vi "GetDevices.vi"(8 "error in (no error)":errorcluster, 11 "service":refnum<class "IcmMessageService.lvclass">) -> (0 "error out":errorcluster, 3 "Body":T1)   [LabVIEW 2016]
doc: "Queries for all equipment asset nodes, which means they have operating states."
uses:
  <vilib>/addons/InsightCM/MessageBus/MessageService/IcmMessageService.lvclass
  <vilib>/addons/InsightCM/MessageBus/Base/controls/KeyValuePair.ctl
  <vilib>/addons/InsightCM/MessageBus/Base/controls/DataGroup.ctl
  <vilib>/addons/InsightCM/MessageBus/Base/controls/DeviceState.ctl
  <vilib>/addons/InsightCM/MessageBus/Base/controls/Condition.ctl
  <vilib>/addons/InsightCM/MessageBus/Base/controls/Trigger.ctl
  <vilib>/addons/InsightCM/MessageBus/Base/controls/BurstModeTrigger.ctl
  <vilib>/addons/InsightCM/MessageBus/Base/controls/Device.ctl
  <vilib>/addons/InsightCM/MessageBus/MessageLibrary/AssetManager/controls/AssetMgrGetDeviceListResponseBody.ctl
panel:
  out "string":string
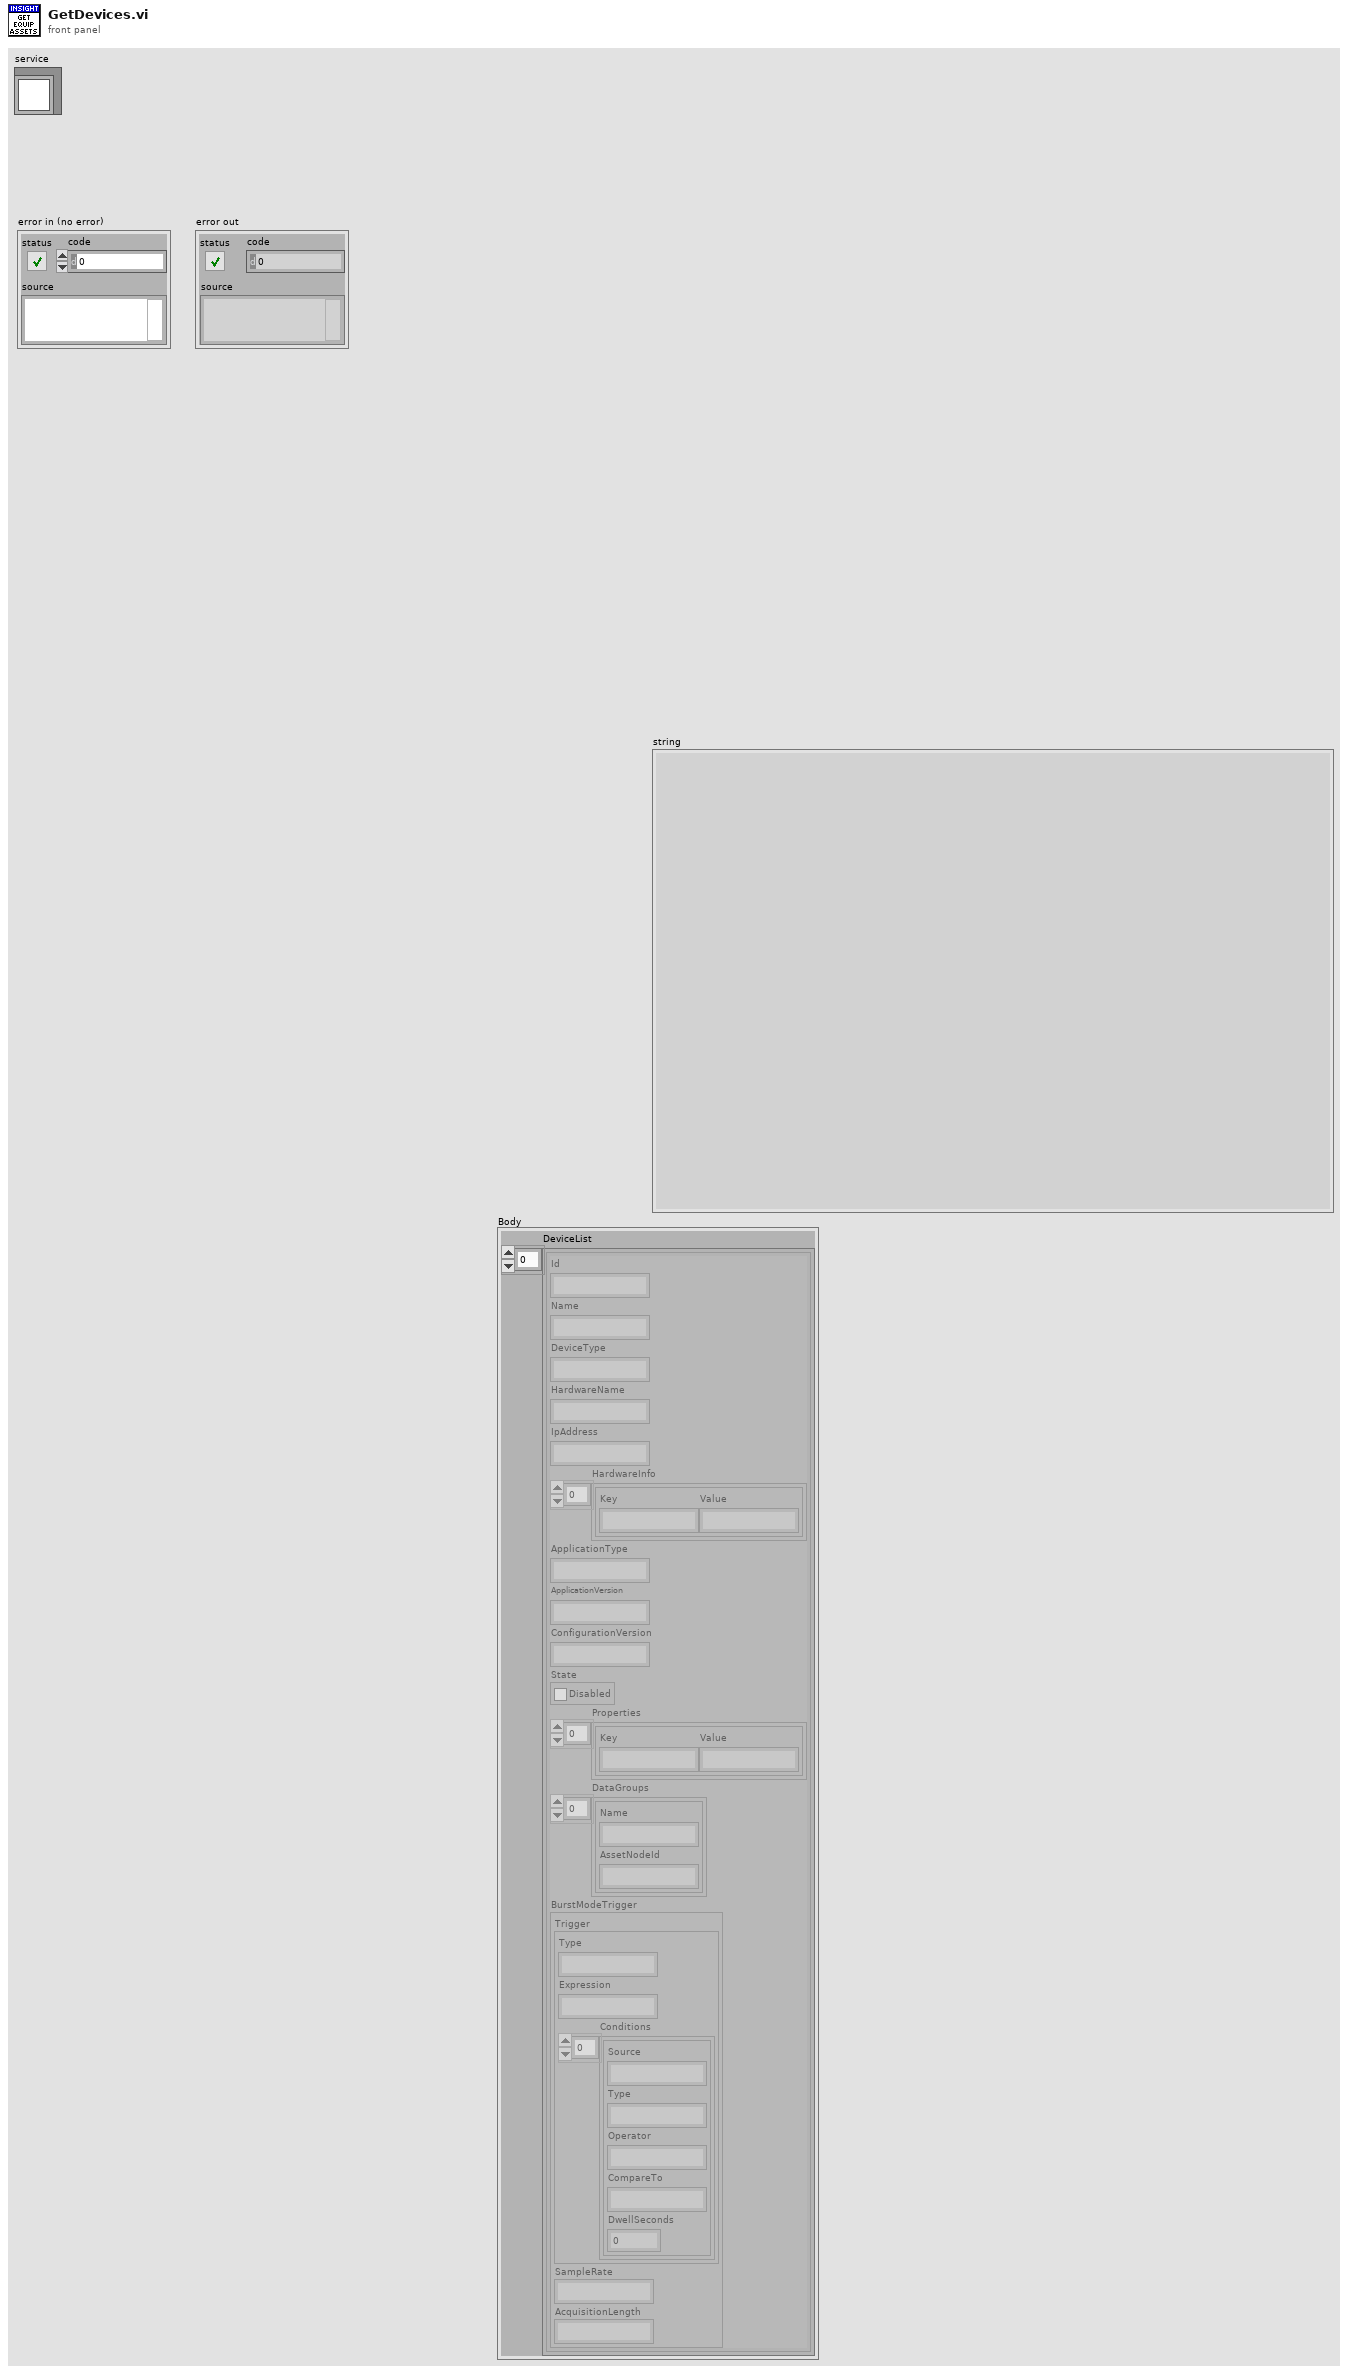
[diagram p1: front panel]
types:
  T1 = typedef "AssetMgrGetDeviceListResponseBody.ctl" = cluster{"DeviceList":T2[]}
  T2 = typedef "Device.ctl" = cluster{"Id":string, "Name":string, "DeviceType":string, "HardwareName":string, "IpAddress":string, "HardwareInfo":T3[], "ApplicationType":string, "ApplicationVersion":string, "ConfigurationVersion":string, "State":T4, "Properties":T3[], "DataGroups":T5[], "BurstModeTrigger":T6}
  T3 = typedef "KeyValuePair.ctl" = cluster{"Key":string, "Value":string}
  T4 = typedef "DeviceState.ctl" = cluster{"Disabled":bool}
  T5 = typedef "DataGroup.ctl" = cluster{"Name":string, "AssetNodeId":string}
  T6 = typedef "BurstModeTrigger.ctl" = cluster{"Trigger":T7, "SampleRate":string, "AcquisitionLength":string}
  T7 = typedef "Trigger.ctl" = cluster{"Type":string, "Expression":string, "Conditions":T8[]}
  T8 = typedef "Condition.ctl" = cluster{"Source":string, "Type":string, "Operator":string, "CompareTo":string, "DwellSeconds":dbl}
  T9 = typedef "Message.ctl" = cluster{"Header":T10, "Body":u8[]}
  T10 = typedef "MessageHeader.ctl" = cluster{"MessageName":string, "Timestamp":i64, "CorrelationId":string, "ContentType":string, "RoutingKey":string, "Properties":T3[]}
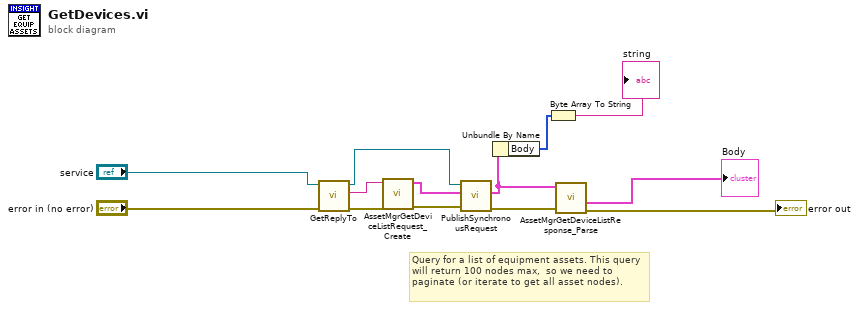
[diagram p0: block diagram]
diagram:
  # "Query for a list of equipment assets. This query will return 100 nodes max,  so we need to paginate (or iterate to get all asset nodes)."
  n1 = call <vilib>:"GetReplyTo.vi"("error in (no error)"="error in (no error)", "service in"="service") -> ("error out"=w9:errorcluster, "reply to"=w10:string, "service out"=w11:refnum<class "IcmMessageService.lvclass">)  [unwired: 7 in]
  n2 = call <vilib>:"AssetMgrGetDeviceListRequest_Create.vi"("error in (no error)"=w9, "ReplyTo"=w10) -> ("error out"=w8:errorcluster, "Message"=w7:T9)  [unwired: 8 in]
  n3 = call <vilib>:"PublishSynchronousRequest.vi"("error in (no error)"=w8, "request"=w7, "service in"=w11) -> ("error out"=w4:errorcluster, "response"=w3:T9)  [unwired: 6 in, 1 out]
  n4 = Unbundle By Name(w3) -> ("Body"=w6:u8[])
  n5 = Byte Array To String(unsigned byte array=w6) -> (string=→"string":string)
  n6 = call <vilib>:"AssetMgrGetDeviceListResponse_Parse.vi"("error in (no error)"=w4, "Message"=w3) -> ("error out"=→"error out":errorcluster, "Body"=→"Body":T1)  [unwired: 6 in, 2 out]
